vi "Run Stimulus Profile.vi"(8 "uutSerialNumber":string, 9 "gatewayIP":string, 10 "file":string, 11 "Sequence Context In":refnum<k7>) -> (0 "error out":errorcluster)   [LabVIEW 2013, in "RTSequenceVIs.lvlib"]
uses:
  RTSequenceVIs.lvlib
  NationalInstruments.VeriStand.RealTimeSequenceDefinitionApi
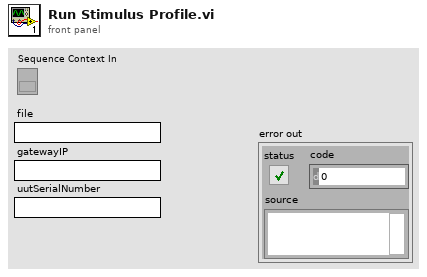
[diagram p1: front panel]
types:
  T1 = typedef "TestStand - Status Monitor.ctl" = cluster{"Sequence Context":refnum<k7>, "Execution":refnum<k7>, "Termination Monitor":refnum<k7>}
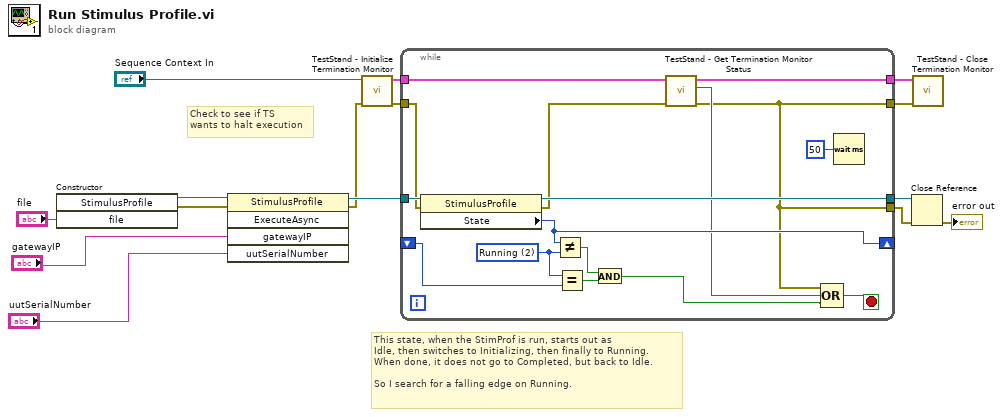
[diagram p0: block diagram]
diagram:
  # "Check to see if TS \nwants to halt execution"
  # "This state, when the StimProf is run, starts out as \nIdle, then switches to Initializing, then finally to Running.\nWhen done, it does not go to Completed, but back to Idle.\n\nSo I search for a falling edge on Running."
  n1 = constructor class="StimulusProfile"("file"="file") -> (reference out=w15:refnum<k24>, error out=w14:errorcluster)  [unwired: 3 in, 2 out]
  n2 = invoke class="StimulusProfile" method="ExecuteAsync"(reference=w15, error in=w14, "gatewayIP"="gatewayIP", "uutSerialNumber"="uutSerialNumber") -> (reference out=w10:refnum<k24>, error out=w1:errorcluster)  [unwired: 1 in, 3 out]
  n3 = call <vilib>:"TestStand - Initialize Termination Monitor.vi"("error in (no error)"=w1, "Sequence Context In"="Sequence Context In") -> ("error out"=w2:errorcluster, "Status Monitor Out"=w5:T1)  [unwired: 8 in]
  n4 = while {
    tunnel: w10 -> [w31]
    tunnel: [w29] -> w9
    tunnel: [w16] -> w8
    shift-right: [w28] -> _
    shift-left: _ -> [w26]
    tunnel: w5 -> [w21]
    tunnel: [w20] -> w4
    tunnel: [w16] -> w3
    tunnel: w2 -> [w18]
    stop <- w22 stop-if-true
    w27 = 2 items=["Idle", "Initializing", "Running", "Paused", "Finalizing", "Complete"] ("State")
    n5 = property class="StimulusProfile"(reference=w31, error in=w18) -> (reference out=w29:refnum<k24>, error out=w19:errorcluster, "State"=w28:i32)
    n6 = Not Equal?(x=w28, y=w27) -> (x != y?=w25:bool)
    n7 = Equal?(x=w27, y=w26) -> (x = y?=w24:bool)
    n8 = And(x=w25, y=w24) -> (x .and. y?=w23:bool)
    n9 = call <vilib>:"TestStand - Get Termination Monitor Status.vi"("error in (no error)"=w19, "Status Monitor In"=w21) -> ("error out"=w16:errorcluster, "Terminating or Aborting"=w17:bool, "Status Monitor Out"=w20:T1)  [unwired: 7 in]
    n10 = Compound Arithmetic op=OR(w16, w17, w23) -> (w22:bool)
    n11 = Wait (ms)(milliseconds to wait=u32 50) -> ()  [unwired: 1 out]
  }
  n12 = Close Reference(reference=w9, error in (no error)=w8) -> (error out=→"error out":errorcluster)
  n13 = call <vilib>:"TestStand - Close Termination Monitor.vi"("error in (no error)"=w3, "Status Monitor In"=w4) -> ()  [unwired: 9 in, 1 out]
